vi "USER-PWD-DB.vi"(5 "Password":string, 7 "Login":string) -> (1 "Verified?":bool)   [LabVIEW 2022 SP3]
doc: "This subi checks if the user login and password are part of a predefined table in order to verify if the user is valid. This subvi is used on the Login Dialog.vi example"
panel:
  in  "Users Table":string[][](table)=[["Operator 1", "Test"], ["Operator 2", "Test"], ["Operator 3", "Test"]]
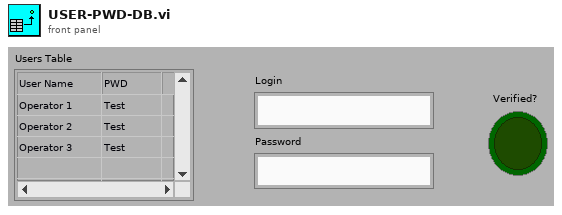
[diagram p1: front panel]
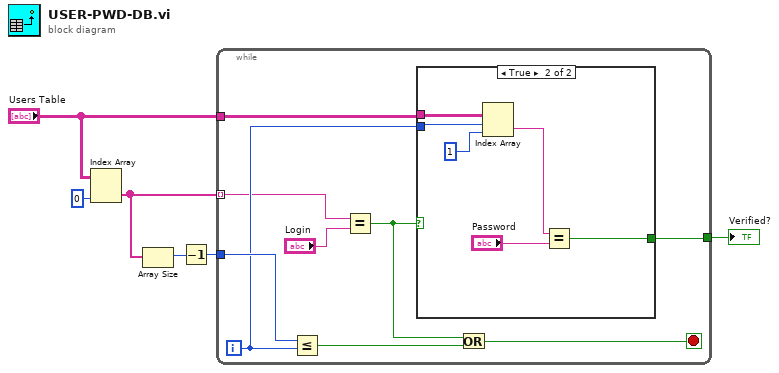
[diagram p0: block diagram]
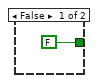
[diagram p2: hidden frame]
diagram:
  n1 = Index Array(array="Users Table", index (col)=0 ("disabled index (col)")) -> (element=w4:string[])  [unwired: 1 in]
  n2 = Array Size(array=w4) -> (size(s)=w5:i32)
  n3 = Decrement(x=w5) -> (x-1=w3:i32)
  n4 = while {
    tunnel: "Users Table" -> [w14]
    tunnel: w4 -> [w11] mode=indexing
    tunnel: w3 -> [w15]
    tunnel: [w10] -> w2
    i -> [w13]
    stop <- w9 stop-if-true
    n5 = Less Or Equal?(x=w15, y=w13) -> (x <= y?=w7:bool)
    n6 = Equal?(x=w11, y="Login") -> (x = y?=w8:bool)
    n7 = case shown="True" w8 {
      tunnel: w14 -> [_ w22]
      tunnel: w13 -> [_ w20]
      tunnel: [FALSE w17] -> w10
      frame False {
      }
      frame True {
        n8 = Index Array(array=w22, index (row)=w20, index (col)=1 ("disabled index (col)")) -> (element=w19:string)
        n9 = Equal?(x=w19, y="Password") -> (x = y?=w17:bool)
      }
    }
    n10 = Or(x=w8, y=w7) -> (x .or. y?=w9:bool)
  }
  "Verified?" <- w2
